vi "Dashboard Main.vi"() -> ()   [LabVIEW 2014]
uses:
  <vilib>/event_ctls.llb/eventvkey.ctl
  <vilib>/Rock Robotics/WPI/Dashboard/WPI_DashboardLogging Global.vi
  <vilib>/Utility/config.llb/Write Key (String).vi
  <vilib>/Utility/config.llb/Write Key (I32).vi
  <vilib>/Utility/file.llb/Write To Spreadsheet File (DBL).vi
  <vilib>/Utility/config.llb/NI_LVConfig.lvlib
panel:
  out "Camera Image 2":T1(plugin-control)
  in  "TCP":refnum<k5>
  in  "Vision":u16(ring) items=["Camera Off", "USB Camera SW", "USB Camera HW", "IP Camera"]
  out "Image Message":string="Timeout in Camera Communications"
  in  "Dashboard Tab":T2(tab)
  in  "DUD CAM":T3={"Frame Rate"=30, "Compression"=30, "Size"=1} {"Frame Rate" scale=1.0..30.0; "Size" items=["640x480", "320x240", "160x120"]}
  out "MotorChart R":cluster{"Numeric":dbl, "Numeric":dbl}(graph)
  out "MotorChart L":T4(graph)
  out "MotorSliders R":cluster{"MotorSlide1":dbl, "MotorSlide2":dbl} {"MotorSlide2" scale=-1.0..1.0 scale format="%#_2e"; "MotorSlide1" scale=-1.0..1.0 scale format="%#_2e"}
  out "MotorSliders L":T5 {"MotorSlide4 2" scale=0.0..14.0 scale format="%#_2e"; "MotorSlide2" scale=-1.0..1.0 scale format="%#_2e"; "MotorSlide1" scale=-1.0..1.0 scale format="%#_2e"}
  out "Gyro":dbl(knob) scale=0.0..360.0
  out "JS1 Z":dbl(slide) scale=-1.0..1.0 scale format="%#_2e"
  out "JS1 Graph":cluster{"X":dbl, "Y":dbl}[](graph)
  out "JS1 Buttons":T6
  out "JS2 Z":dbl(slide) scale=-1.0..1.0 scale format="%#_2e"
  out "JS2 Graph":cluster{"X":dbl, "Y":dbl}[](graph)
  out "JS2 Buttons":T6
  out "Mode":T7(ring)=enum."Auto Disabled"
  in  "DB Camera Config":bool
  in  "Big Cam":T3={"Frame Rate"=30, "Compression"=30, "Size"=1} {"Frame Rate" scale=1.0..30.0; "Size" items=["640x480", "320x240", "160x120"]}
  in  "Small Cam":T3={"Frame Rate"=30, "Compression"=30, "Size"=1} {"Frame Rate" scale=1.0..30.0; "Size" items=["640x480", "320x240", "160x120"]}
  in  "CamPow":bool
  in  "Toggle View":bool
  in  "Rec Mode":enum32{"Stop", "Record", "Playback"}(radio)
  out "Mbps 2":bool
  out "Mbps":dbl format="%#.1g"
  out "fps":dbl format="%#.1g"
  out "Mbps 4":bool
  out "Mbps 3":dbl format="%#.1g"
  out "fps 2":dbl format="%#.1g"
  out "Camera Addr":string
  in  "DB/String 9":string
  in  "DB/String 8":string
  in  "DB/String 7":string
  in  "DB/String 6":string
  in  "DB/String 5":string
  in  "DB/String 4":string
  in  "DB/String 3":string
  in  "DB/String 2":string
  in  "DB/String 1":string
  in  "DB/String 0":string
  in  "DB/Slider 0":dbl(slide) scale=0.0..5.0
  in  "DB/Slider 1":dbl(slide) scale=0.0..5.0
  in  "DB/Slider 2":dbl(slide) scale=0.0..5.0
  in  "DB/Slider 3":dbl(slide) scale=0.0..5.0
  out "DB/LED 3":bool
  out "DB/LED 2":bool
  out "DB/LED 1":bool
  out "DB/LED 0":bool
  in  "DB/Button 3":bool
  in  "DB/Button 2":bool
  in  "DB/Button 1":bool
  in  "DB/Button 0":bool caption="New Name"
  in  "Elevator Go":bool
  in  "Elevator Height":sgl(slide) step=1 scale=0.0..5.0 scale format="%#1.1g"
  in  "Sub Tote":bool
  in  "Add Tote":bool
  out "Tote Count":dbl
  in  "Manual Control":bool
  in  "Winch Cim 2":dbl(slide) scale=-1.0..1.0
  in  "Winch Cim 1":dbl(slide) scale=-1.0..1.0
  in  "Ejector Motor":dbl(slide) scale=-1.0..1.0
  in  "End Effector Motor 1":dbl(slide) scale=-1.0..1.0
  in  "End Effector Motor 2":dbl(slide) scale=-1.0..1.0
  in  "Left Drive Motor":dbl(slide) scale=-1.0..1.0
  in  "Right Drive Motor":dbl(slide) scale=-1.0..1.0
  in  "Test Slider":dbl(slide) scale=0.0..100.0 scale format="%#_3g"
  in  "On/Off":bool caption="Solenoid"
  in  "Test Name":u16(ring) items=["Select the test to run...", "Example Test", "-------------------------------", "List of tests is built in robot code.", "Replace with your own automated tests."]
  in  "Test Tree":string(tree)
  in  "Motor":cluster{"Value":dbl, "Enable":bool} {"Value" scale=-1.0..1.0 scale format="%#_3g"}
  out "Progress":T8 {"Test Progress" scale=0.0..100.0}
  in  "Rev/Fwd":cluster{"Forward":bool, "Reverse":bool}
  in  "Test Ring":u16(ring) items=["Monochrome", "Color"]
  in  "Listbox":i32(listbox)
  out "Tree":string(tree)
  in  "Save To":path
  in  "Export To File":bool
  out "Camera Image":T1(plugin-control)
  out "Boolean":bool
  # "Left"
  # "Front"
  # "Right"
  # "Battery"
  # "Big Cam"
  # "Small Cam"
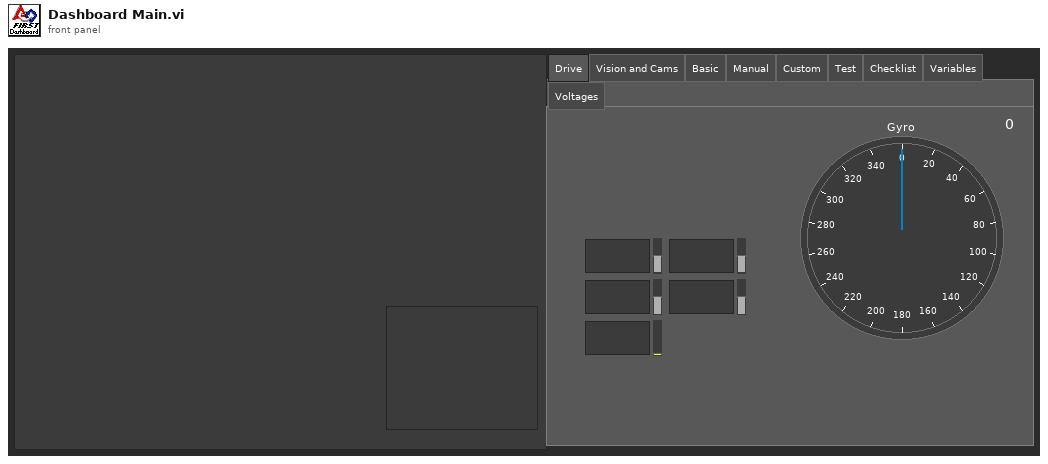
[diagram p1: front panel]
types:
  T1 = typedef "IMAQ Image.ctl" = refnum<image>
  T2 = enum32{"Drive", "Vision and Cams", "Basic", "Manual", "Custom", "Test", "Checklist", "Variables", "Voltages"}
  T3 = cluster{"Frame Rate":i32, "Compression":i32, "Size":u16}
  T4 = cluster{"Numeric":dbl, "Numeric":dbl, "Battery V":dbl}
  T5 = cluster{"MotorSlide1":dbl, "MotorSlide2":dbl, "MotorSlide4 2":dbl}
  T6 = cluster{bool, bool, bool, bool, bool, bool, bool, bool, bool, bool, bool, bool}
  T7 = enum8{"Tele-Op Disabled", "Tele-Op Enabled", "Auto Disabled", "Auto Enabled", "Test Disabled", "Test Enabled", "Disconnected", "No Code", "E-Stop"}
  T8 = cluster{"Test Progress":u8, "Test Progress Text":string}
  T9 = typedef "Image Type" = u32
  T10 = enum32{"Drive", "Basic", "Custom", "Test", "Checklist", "Variables"}
  T11 = cluster{"Camera Image":refnum<vi>, "Dashboard Tab":refnum<vi>, "Boolean":refnum<vi>, "Vision":refnum<vi>, "Rec Mode":refnum<vi>, "Test Slider":refnum<vi>, "On/Off ":refnum<vi>, "Test Ring":refnum<vi>, "Rev/Fwd":refnum<vi>, "Test Name":refnum<vi>, "Motor":refnum<vi>, "Progress":refnum<vi>, "CheckList":refnum<vi>, "Tree":refnum<vi>, "Test Tree":refnum<vi>}
  T12 = cluster{"Error Strings":string, "Disable Counts":cluster{u16, u16}, "Rail Faults":cluster{u16, u16, u16}, "Robot IP":string, "DB Mode":u8, "Event Info":cluster{"Name":string, "Type":u8, "Number":u16, "Replay":u8}, "Camera Addr":string}
  T13 = cluster{"Storage":cluster{"Disk Free":u64, "RAM Block":u32, "RAM free":u32}, "CPU Utilization":cluster{"CPU % ISR":sgl, "CPU % Time Crit":sgl, "CPU % Timed Str":sgl, "CPU % High":sgl, "CPU % Above":sgl, "CPU % Normal":sgl, "CPU % Low":sgl}, "CAN":cluster{"% Bus Utilization":sgl, "Bus Off Cnt":u32, "TX_FIFO Full Cnt":u32, "Receive Error Cnt":u8, "Transmit Error Cnt":u8}, "HID":cluster{"HID Outputs":u32, "Rumble Low":u16, "Rumble High":u16}[]}
  T14 = cluster{"Status bits":cluster{"Test Mode":bool, "Autonomous":bool, "Enabled":bool, "Code Start":bool, "Brownout":bool, "Reserved 2":bool, "Reserved 3":bool, "E-Stop":bool}, "Code Trace":cluster{"Disabled":bool, "TeleOp":bool, "Auto":bool, "Test":bool}, "Controller Type":enum16{"unknown", "cRIO", "roboRio"}, "Code?":enum16{"unknown", "noCode", "code"}, "Battery V":dbl}
  T15 = cluster{"Control Bits":cluster{"TestMode":bool, "Autonomous":bool, "Enabled":bool, "FMS Present":bool, bool, bool, bool, "E-Stop":bool}, "Team Station ":u8, "Countdown":sgl, "Joystick Values":cluster{"Axes":dbl[], "Buttons":bool[], "POVs":i16[]}[]}
  T16 = cluster{"Axes":dbl[], "Buttons":bool[], "POVs":i16[]}[]
  T17 = cluster{"Axes":dbl[], "Buttons":bool[], "POVs":i16[]}
  T18 = cluster{"Buttons[0]":bool, "Buttons[1]":bool, "Buttons[2]":bool, "Buttons[3]":bool, "Buttons[4]":bool, "Buttons[5]":bool, "Buttons[6]":bool, "Buttons[7]":bool, "Buttons[8]":bool, "Buttons[9]":bool, "Buttons[10]":bool, "Buttons[11]":bool}
  T19 = typedef "NI_LVConfig.lvlib/Config Data RefNum.ctl" = refnum<k1>
  T20 = cluster{"Operation":enum16{"Update", "Clear"}, "Color Box":u32}[]
  T21 = typedef "eventvkey.ctl" = enum16{"ASCII", "Enter", "Return", "Shift", "Ctrl", "Alt", "Cmd", "Opt", "Caps", "NumLock", "Clear", "Break", "Up", "Down", "Left", "Right", "Insert", "Delete", "Home", "End", "PageUp", "PageDown", "Escape", "Help", "Pause", "ScrollLock", "F1", "F2", "F3", "F4", "F5", "F6", "F7", "F8", "F9", "F10", "F11", "F12", "F13", "F14", "F15", "F16", "F17", "F18", "F19", "F20", "F21", "F22", "F23", "F24", "Play", "VolumeUp", "VolumeDown", "Mute", "Two Byte Char"}
  T22 = cluster{"Image Size":bool, "Image Type":bool, "Pixel Value":bool, "ROI Information":bool, "Zoom Factor":bool}
  T23 = enum8{"Enabled", "Disabled", "Disabled and Grayed Out"}
  T24 = cluster{"Operation":enum16{"Update", "Clear"}, "Color Box":u32}
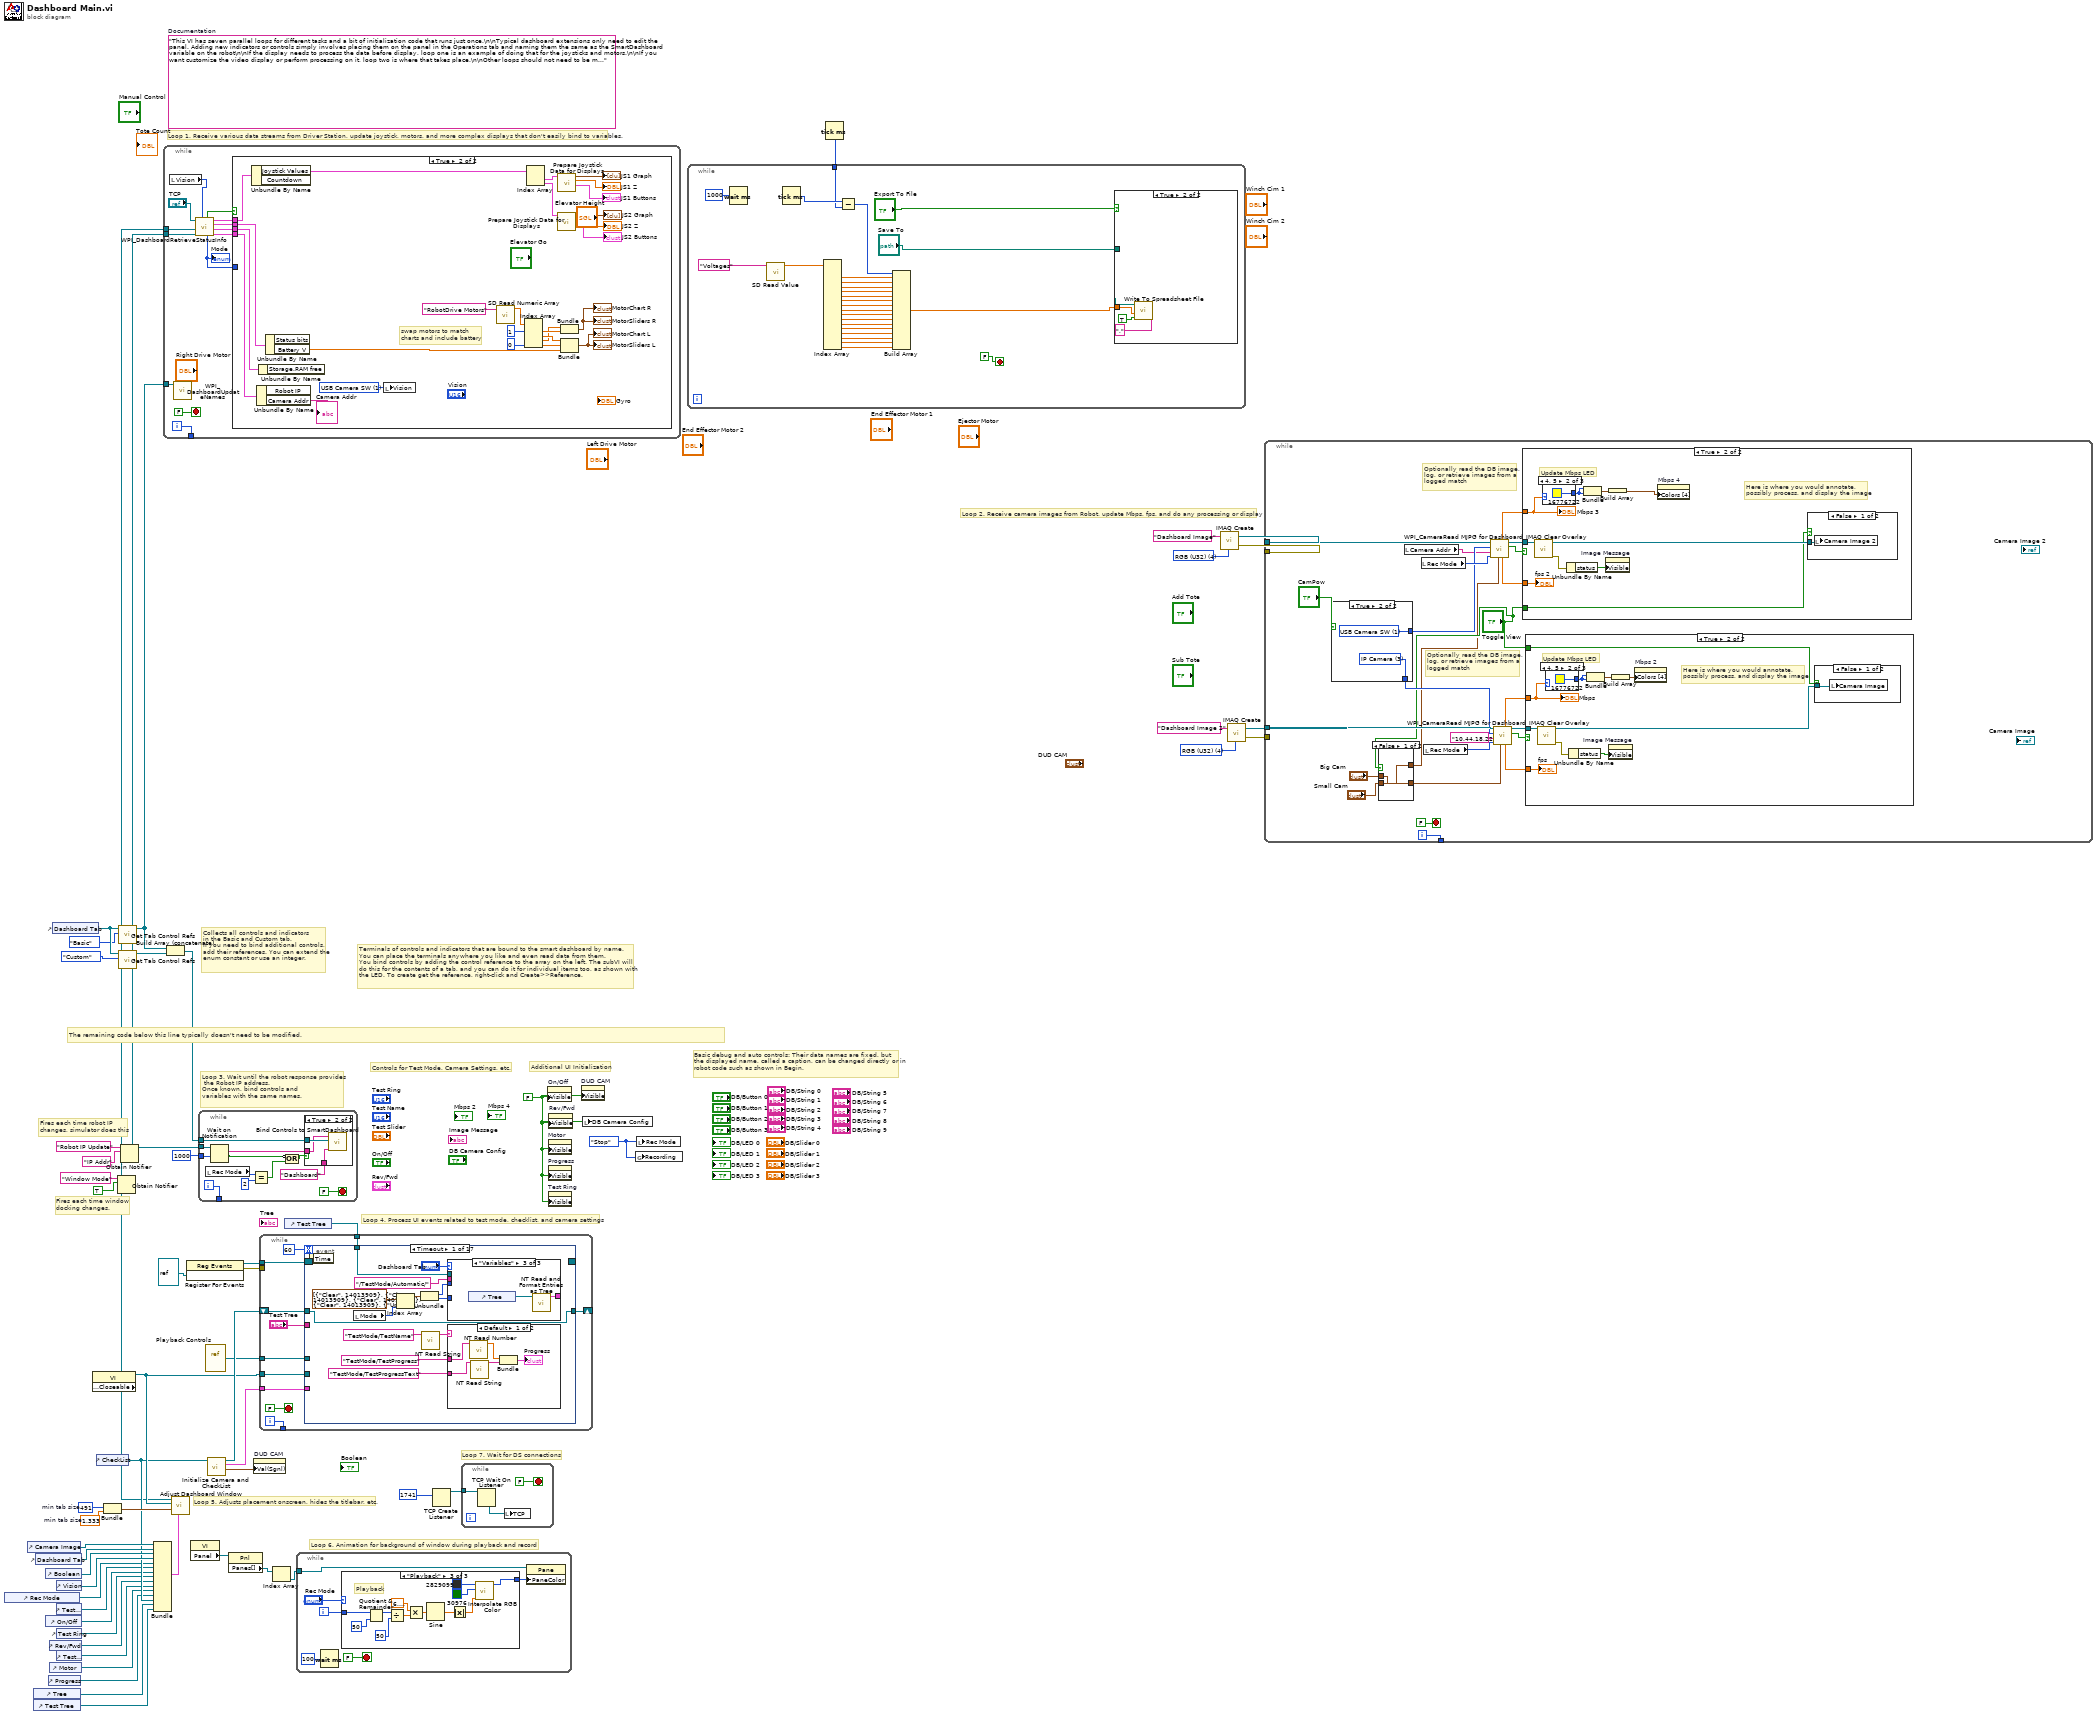
[diagram p0: block diagram]
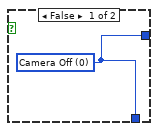
[diagram p3: hidden frame]
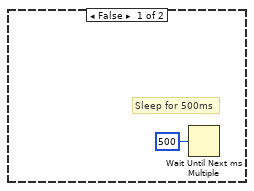
[diagram p4: hidden frame]
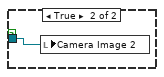
[diagram p5: hidden frame]
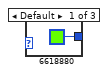
[diagram p6: hidden frame]
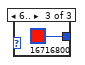
[diagram p7: hidden frame]
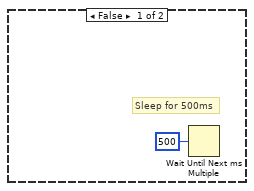
[diagram p8: hidden frame]
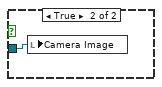
[diagram p9: hidden frame]
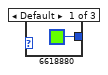
[diagram p10: hidden frame]
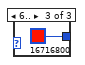
[diagram p11: hidden frame]
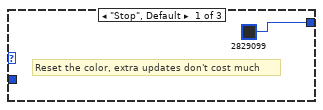
[diagram p14: hidden frame]
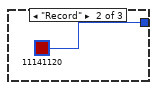
[diagram p15: hidden frame]
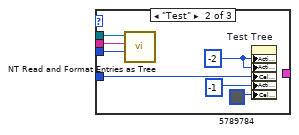
[diagram p18: hidden frame]
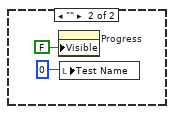
[diagram p19: hidden frame]
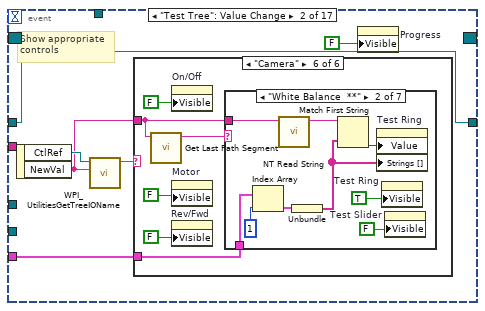
[diagram p20: hidden frame]
diagram:
  w7 = T9 4 items=["Grayscale (U8)", "Grayscale (I16)", "Grayscale (SGL)", "Complex (CSG)", "RGB (U32)", "HSL (U32)", "RGB (U64)"] ("Image Type")
  w32 = 491  # min tab size
  w31 = 1.333  # min tab size
  w3 = enum32{"Stop", "Record", "Playback"}."Stop" ("Rec Mode")
  w14 = FALSE ("Visible")
  (unwired) "This VI has seven parallel loops for different tasks and a bit of initialization code that runs just once.\n\nTypical dashboard extensions only need to edit the panel. Adding new indicators or controls simply involves placing them on the panel in the Operations tab and naming them the same as the SmartDashboard variable on the robot\n\nIf the display needs to process the data before display, loop one is an example of doing that for the joysticks and motors.\n\nIf you want customize the video display or perform processing on it, loop two is where that takes place.\n\nOther loops should not need to be modified. They are pretty standard, and document the task they perform."  # Documentation
  w57 = T9 4 items=["Grayscale (U8)", "Grayscale (I16)", "Grayscale (SGL)", "Complex (CSG)", "RGB (U32)", "HSL (U32)", "RGB (U64)"] ("Image Type")
  # "Loop 7. Wait for DS connections"
  # "Basic debug and auto controls: Their data names are fixed, but\nthe displayed name, called a caption, can be changed directly or in\nrobot code such as shown in Begin."
  # "Controls for Test Mode, Camera Settings, etc."
  # "Additional UI Initialization"
  # "Loop 6. Animation for background of window during playback and record"
  # "Fires each time robot IP\nchanges, simulator does this"
  # "Fires each time window\ndocking changes."
  # "Collects all controls and indicators\nin the Basic and Custom tab.\nIf you need to bind additional controls,\nadd their references. You can extend the\nenum constant or use an integer."
  # "The remaining code below this line typically doesn't need to be modified."
  # "Loop 4. Process UI events related to test mode, checklist, and camera settings"
  # "Terminals of controls and indicators that are bound to the smart dashboard by name.\nYou can place the terminals anywhere you like and even read data from them.\nYou bind controls by adding the control reference to the array on the left. The subVI will\ndo this for the contents of a tab, and you can do it for individual items too, as shown with\nthe LED. To create get the reference, right-click and Create>>Reference."
  # "Loop 3. Wait until the robot response provides\n the Robot IP address.\nOnce known, bind controls and\nvariables with the same names."
  # "Loop 5. Adjusts placement onscreen, hides the titlebar, etc."
  # "Loop 1. Receive various data streams from Driver Station, update joystick, motors, and more complex displays that don't easily bind to variables."
  # "Loop 2. Receive camera images from Robot, update Mbps, fps, and do any processing or display"
  n1 = control-ref of="Rec Mode"() -> (w20:refnum<vi>)
  n2 = control-ref of="Camera Image"() -> (w35:refnum<vi>)
  n3 = control-ref of="Tree"() -> (w24:refnum<vi>)
  n4 = control-ref of="Test Tree"() -> (w23:refnum<vi>)
  n5 = control-ref of="Dashboard Tab"() -> (w34:refnum<vi>)
  n6 = control-ref of="Boolean"() -> (w29:refnum<vi>)
  n7 = control-ref of="On/Off"() -> (w18:refnum<vi>)
  n8 = control-ref of="Progress"() -> (w15:refnum<vi>)
  n9 = control-ref of="Rev/Fwd"() -> (w16:refnum<vi>)
  n10 = control-ref of="Motor"() -> (w21:refnum<vi>)
  n11 = control-ref of="Dashboard Tab"() -> (w38:refnum<vi>)
  n12 = control-ref of="Test Slider"() -> (w19:refnum<vi>)
  n13 = control-ref of="Vision"() -> (w33:refnum<vi>)
  n14 = control-ref of="Test Ring"() -> (w17:refnum<vi>)
  n15 = control-ref of="Test Name"() -> (w22:refnum<vi>)
  n16 = property class="VI" props=["Front Panel.Closeable"]() -> (reference out=w39:refnum<vi>)  [unwired: 2 in, 2 out]
  n17 = control-ref of="CheckList"() -> (w25:refnum<vi>)
  n18 = Bundle("min tab size"=w32, "min tab size"=w31) -> (w30:cluster{"min tab size":i32, "min tab size":dbl})  [unwired: 1 in]
  n19 = Obtain Notifier(name (unnamed)="Window Mode", notification data type=TRUE) -> (notifier out=w11:refnum<notifier>)  [unwired: 2 in, 2 out]
  n20 = call <vilib>:"Get Tab Control Refs.vi"("Page Index"=T10."Basic" ("Dashboard Tab"), "TabControl in"=w38) -> ("ControlsOnPage"=w12:refnum<vi>[])  [unwired: 9 in]
  n21 = call <vilib>:"Get Tab Control Refs.vi"("Page Index"=T10."Custom" ("Dashboard Tab"), "TabControl in"=w38) -> ("ControlsOnPage"=w37:refnum<vi>[])  [unwired: 9 in]
  n22 = Obtain Notifier(name (unnamed)="Robot IP Update", notification data type="IP Addr" ("name (unnamed)")) -> (notifier out=w13:refnum<notifier>)  [unwired: 2 in, 2 out]
  n23 = Bundle("Camera Image"=w35, "Dashboard Tab"=w34, "Boolean"=w29, "Vision"=w33, "Rec Mode"=w20, "Test Slider"=w19, "On/Off"=w18, "Test Ring"=w17, "Rev/Fwd"=w16, "Test Name"=w22, "Motor"=w21, "Progress"=w15, "CheckList"=w25, "Tree"=w24, "Test Tree"=w23) -> (w26:T11)  [unwired: 1 in]
  n24 = while {
    tunnel: [w69] -> _
    tunnel: w13 -> [w63]
    tunnel: w12 -> [w62]
    tunnel: w11 -> [w58]
    i -> [w69]
    stop <- FALSE stop-if-true
    n25 = local read "Vision"() -> (w60:u16)
    n26 = call <vilib>:"WPI_DashboardUpdateNames.vi"("Controls on Tab"=w62) -> ()  [unwired: 11 in]
    n27 = call <vilib>:"WPI_DashboardRetrieveStatusInfo.vi"("Vision"=w60, "Binding Refnum"=w63, "Window Mode Notifier"=w58, "TCP Cnx"="TCP") -> ("Power and Errors"=w64:T12, "Robot Metrics"=w67:T13, "Status Info"=w68:T14, "Control Info"=w65:T15, "Robot Mode"=w61:T7, "Process?"=w66:bool)  [unwired: 2 in]
    "Mode" <- w61
    n28 = case shown="True" w66 {
      tunnel: w68 -> [_ w96]
      tunnel: w67 -> [_ w95]
      tunnel: w65 -> [_ w94]
      tunnel: w64 -> [_ w93]
      tunnel: w61 -> [_ _]
      frame False {
      }
      frame True {
        w72 = u16 1 items=["Camera Off", "USB Camera SW", "USB Camera HW", "IP Camera"] ("Vision")
        # "swap motors to match\ncharts and include battery"
        n29 = Unbundle By Name(w94) -> ("Joystick Values"=w81:T16)  [unwired: 1 out]
        n30 = Unbundle By Name(w93) -> ("Camera Addr"=→"Camera Addr":string)  [unwired: 1 out]
        n31 = Unbundle By Name(w95) -> ()  [unwired: 1 out]
        n32 = Unbundle By Name(w96) -> ("Battery V"=w82:dbl)  [unwired: 1 out]
        n33 = local write "Vision"(w72) -> ()
        n34 = call <vilib>:"SD Read Numeric Array.vi"("Name"="RobotDrive Motors") -> ("Numeric Array"=w84:dbl[])  [unwired: 8 in, 2 out]
        n35 = Index Array(array=w84, index #1=1, index #4=0) -> (element #1=w88:dbl, element #2=w89:dbl, element #3=w87:dbl, element #4=w92:dbl)  [unwired: 2 in]
        n36 = Index Array(array=w81) -> (element #1=w80:T17, element #2=w76:T17)  [unwired: 2 in]
        n37 = call "Prepare Joystick Data for Displays.vi"("Joystick Values"=w76) -> ("Buttons"=→"JS2 Buttons":T18, "Z Axis"=→"JS2 Z":dbl, "Cartesian Data"=→"JS2 Graph":cluster{"X axis":dbl, "X axis":dbl}[])  [unwired: 8 in]
        n38 = call "Prepare Joystick Data for Displays.vi"("Joystick Values"=w80) -> ("Buttons"=→"JS1 Buttons":T18, "Z Axis"=→"JS1 Z":dbl, "Cartesian Data"=→"JS1 Graph":cluster{"X axis":dbl, "X axis":dbl}[])  [unwired: 8 in]
        n39 = Bundle("Numeric"=w87, "Numeric"=w88) -> (→"MotorChart R" →"MotorSliders R":cluster{"Numeric":dbl, "Numeric":dbl})  [unwired: 1 in]
        n40 = Bundle("Numeric"=w89, "Numeric"=w92, "Battery V"=w82) -> (→"MotorChart L" →"MotorSliders L":T4)  [unwired: 1 in]
      }
    }
  }
  n41 = Build Array (concatenate)(w12, w37) -> (w36:refnum<vi>[])
  n42 = call "Adjust Dashboard Window.vi"("Sizing Refnums"=w26, "Size Constraints"=w30, "VI"=w39, "Notifier in"=w11) -> ()  [unwired: 8 in]
  n43 = register-events(refnum<vi> refnum) -> (reference out=w43:refnum<event-registration>, error out=w42:errorcluster)  [unwired: 2 in]
  n44 = property class="VI"() -> ("Panel"=w46:refnum<vi>)  [unwired: 2 in, 2 out]
  n45 = while {
    tunnel: w36 -> [w108]
    tunnel: w13 -> [w106]
    tunnel: [w104] -> _
    tunnel: u32 1000 ("milliseconds to wait") -> [w103]
    i -> [w104]
    stop <- FALSE stop-if-true
    n46 = local read "Rec Mode"() -> (w99:enum32{"Stop", "Record", "Playback"})
    n47 = Wait on Notification(notifier=w106, timeout in ms (-1)=w103) -> (notification=w105:string, timed out?=w101:bool)  [unwired: 2 in, 2 out]
    n48 = Equal?(x=w99, y=u16 2 ("Rec Mode")) -> (x = y?=w100:bool)
    n49 = Compound Arithmetic op=OR(invert w101, w100) -> (w102:bool)
    n50 = case shown="True" w102 {
      tunnel: w108 -> [_ w111]
      tunnel: w105 -> [_ w110]
      tunnel: "Dashboard" -> [_ w109]
      frame False {
      }
      frame True {
        n51 = call <vilib>:"Bind Controls to SmartDashboard.vi"("Client Name"=w109, "Bound Control Refs"=w111, "Server IP Address"=w110) -> ()  [unwired: 9 in]
      }
    }
  }
  n52 = vi-ref "Playback Controls.vi"() -> (w44:refnum<vi>)
  n53 = call "Initialize Camera and CheckList.vi"("ListBox in"=w25) -> ("Cluster"=w50:cluster{"value":i32, "value":i32, "index":i32}, "Array"=w51:cluster{string[]}[], "File Refnum"=w49:T19)  [unwired: 8 in]
  n54 = property class="Pnl"(reference=w46) -> ("Panes[]"=w47:refnum<vi>[])  [unwired: 1 in, 2 out]
  n55 = property on="DUD CAM" class="Clust (strict)"("Val(Sgnl)"=w50) -> ()  [unwired: 2 in, 2 out]
  n56 = Index Array(array=w47) -> (element=w45:refnum<vi>)  [unwired: 1 in]
  n57 = control-ref of="Test Tree"() -> (w48:refnum<vi>)
  n58 = while {
    tunnel: w51 -> [w119]
    shift-right: [w118] -> _
    shift-left: w49 -> [w117]
    tunnel: [w116] -> _
    tunnel: w48 -> [w115]
    tunnel: w44 -> [w114]
    tunnel: w43 -> [w113]
    tunnel: w42 -> [_]
    tunnel: w39 -> [w112]
    i -> [w116]
    stop <- FALSE stop-if-true
    n59 = event shown="[0] Timeout" {
      selector: w113 -> [_ _ _ _ _ _ _ _ _ _ _ _ _ _ _ _ _]
      dyn-events: [_ _ _ _ _ _ _ _ _ _ _ _ _ w357 _ _ _] -> _
      timeout: u32 60 ("milliseconds to wait") -> [_ _ _ _ _ _ _ _ _ _ _ _ _ _ _ _ _]
      tunnel: w115 -> [w131 _ _ _ _ _ _ _ _ _ _ _ _ _ _ _ _]
      tunnel: "Test Tree" -> [_ _ _ _ _ _ _ _ w326 w334 w336 w340 w348 _ _ _ _]
      tunnel: w119 -> [_ w153 _ _ _ _ w290 w320 _ _ _ _ _ _ _ _ _]
      tunnel: [w127 w152 w251 w256 w264 w276 w289 w313 w325 w332 w335 w339 w347 w359 w373 w374 w384] -> w118
      tunnel: w117 -> [w127 w152 w251 w256 w264 w276 w288 w313 w325 w332 w335 w339 w347 w359 w373 w374 w384]
      tunnel: w114 -> [_ _ _ _ _ _ _ _ _ _ _ _ _ w360 _ w377 _]
      tunnel: w112 -> [_ _ _ _ _ _ _ _ _ _ _ _ _ w355 _ _ _]
      event Timeout {
        n60 = event-data() -> ()  [unwired: 1 in, 1 out]
        n61 = local read "Mode"() -> (w130:T7)
        n62 = Index Array(array=T20 [{"Operation"=enum."Clear", "Color Box"=14013909}, {"Operation"=enum."Clear", "Color Box"=14013909}, {"Operation"=enum."Clear", "Color Box"=14013909}, {"Operation"=enum."Clear", "Color Box"=14013909}, {"Operation"=enum."Update", "Color Box"=14013909}, {"Operation"=enum."Update", "Color Box"=16777215}, {"Operation"=enum."Clear", "Color Box"=14013909}, {"Operation"=enum."Clear", "Color Box"=14013909}, {"Operation"=enum."Clear", "Color Box"=14013909}], index=w130) -> (element=w125:T24)
        n63 = Unbundle(w125) -> ("Operation"=w124:enum16{"Update", "Clear"}, "Color Box"=w123:u32)
        n64 = call <vilib>:"NT Read String.vi"("Name"="TestMode/TestName") -> ("String"=w134:string)  [unwired: 9 in, 1 out]
        n65 = case shown="\"Variables\"" "Dashboard Tab" {
          tunnel: w131 -> [_ w142 _]
          tunnel: "/TestMode/Automatic/" ("Name Pattern") -> [_ w141 _]
          tunnel: w124 -> [_ w140 _]
          tunnel: [_ _ w144] -> _
          tunnel: w123 -> [_ w136 _]
          frame "Custom", Default {
          }
          frame "Test" {
            w139 = -2 ("Active Item:Row Number")
            n66 = call <vilib>:"NT Read and Format Entries as Tree.vi"("Operation"=w140, "Name Pattern"=w141, "Tree Refnum"=w142) -> ()  [unwired: 7 in, 2 out]
            n67 = property on="Test Tree" class="Tree (strict)"("Active Item Row Number"=w139, "ActiveColNum"=w139, "CellBG"=w136, "Active Item Row Number"=-1 ("Active Item:Row Number"), "CellBG"=u32 5789784 ("Color Box")) -> ()  [unwired: 2 in, 2 out]
          }
          frame "Variables" {
            n68 = control-ref of="Tree"() -> (w143:refnum<vi>)
            n69 = call <vilib>:"NT Read and Format Entries as Tree.vi"("Tree Refnum"=w143) -> ("Formatted Strings"=w144:cluster{"Name":string, "Value":string}[])  [unwired: 9 in, 1 out]
          }
        }
        n70 = case shown="Default" w134 {
          tunnel: "TestMode/TestProgress" ("Name") -> [w146 _]
          tunnel: "TestMode/TestProgressText" ("Name") -> [w145 _]
          frame Default {
            n71 = call <vilib>:"NT Read Number.vi"("Name"=w146) -> ("Numeric"=w147:dbl)  [unwired: 9 in, 1 out]
            n72 = call <vilib>:"NT Read String.vi"("Name"=w145) -> ("String"=w148:string)  [unwired: 9 in, 1 out]
            n73 = Bundle("Numeric"=w147, "String"=w148) -> (→"Progress":cluster{"Numeric":dbl, "String":string})  [unwired: 1 in]
          }
          frame "" {
            n74 = property on="Progress" class="Clust (strict)"("Visible"=FALSE) -> ()  [unwired: 2 in, 2 out]
            n75 = local write "Test Name"(u16 0) -> ()
          }
        }
      }
      event "Test Tree": Value Change {
        # "Show appropriate\ncontrols"
        n76 = event-data() -> ("CtlRef"=w156:refnum<vi>, "NewVal"=w154:string)  [unwired: 1 in]
        n77 = call <vilib>:"WPI_UtilitiesGetTreeIOName.vi"("NewVal"=w154, "TreeControl in"=w156) -> ("I/O Name"=w157:string)  [unwired: 9 in]
        n78 = case shown="\"Camera\"" w157 {
          selector: w157 -> [_ w164 _ w182 w191 _]
          tunnel: w154 -> [_ _ w179 w181 _ w198]
          tunnel: w153 -> [_ _ _ _ _ w197]
          frame Default {
            w159 = FALSE ("Visible")
            w158 = FALSE ("Visible")
            n79 = property on="Motor" class="Clust (strict)"("Visible"=w158) -> ()  [unwired: 2 in, 2 out]
            n80 = property on="Test Ring" class="Ring (strict)"("Visible"=w158) -> ()  [unwired: 2 in, 2 out]
            n81 = property on="Rev/Fwd" class="Clust (strict)"("Visible"=w159) -> ()  [unwired: 2 in, 2 out]
            n82 = property on="On/Off" class="Bool (strict)"("Visible"=w159) -> ()  [unwired: 2 in, 2 out]
            n83 = property on="Test Slider" class="Slide (strict)"("Visible"=w159) -> ()  [unwired: 2 in, 2 out]
          }
          frame "Motor", "PWM" {
            w165 = FALSE ("Visible")
            n84 = case shown="\"Motor\", Default" w164 {
              tunnel: [1.0 ("Value") -1.0 ("Value")] -> w163
              tunnel: [255.0 ("Value") 1.0 ("Value")] -> w162
              tunnel: [128.0 ("Value") 0.0 ("Value")] -> w161
              tunnel: [64.0 ("Value") 0.5 ("Value")] -> w160
              frame "PWM" {
              }
              frame "Motor", Default {
              }
            }
            n85 = property on="Motor" class="Clust (strict)"("Visible"=TRUE) -> ()  [unwired: 2 in, 2 out]
            n86 = property on="Value" class="Slide (strict)"("Value"=w161, "Scale.Minimum"=w163, "Scale.Maximum"=w162, "Scale.Increment"=w160) -> ()  [unwired: 2 in, 2 out]
            n87 = property on="On/Off" class="Bool (strict)"("Visible"=w165) -> ()  [unwired: 2 in, 2 out]
            n88 = property on="Test Slider" class="Slide (strict)"("Visible"=w165) -> ()  [unwired: 2 in, 2 out]
            n89 = property on="Test Ring" class="Ring (strict)"("Visible"=w165) -> ()  [unwired: 2 in, 2 out]
            n90 = property on="Rev/Fwd" class="Clust (strict)"("Visible"=w165) -> ()  [unwired: 2 in, 2 out]
          }
          frame "Servo" {
            w177 = FALSE ("Visible")
            n91 = call <vilib>:"NT Read Number.vi"("Name"=w179) -> ("Numeric"=w178:dbl)  [unwired: 9 in, 1 out]
            n92 = property on="Test Slider" class="Slide (strict)"("Visible"=TRUE, "Scale.Maximum"=170.0 ("Scale.Range:Maximum")) -> ()  [unwired: 2 in, 2 out]
            n93 = local write "Test Slider"(w178) -> ()
            n94 = property on="Motor" class="Clust (strict)"("Visible"=w177) -> ()  [unwired: 2 in, 2 out]
            n95 = property on="Rev/Fwd" class="Clust (strict)"("Visible"=w177) -> ()  [unwired: 2 in, 2 out]
            n96 = property on="On/Off" class="Bool (strict)"("Visible"=w177) -> ()  [unwired: 2 in, 2 out]
            n97 = property on="Test Ring" class="Ring (strict)"("Visible"=w177) -> ()  [unwired: 2 in, 2 out]
          }
          frame "Relay", "Solenoid" {
            w180 = FALSE ("Visible")
            n98 = property on="Motor" class="Clust (strict)"("Visible"=w180) -> ()  [unwired: 2 in, 2 out]
            n99 = property on="Test Slider" class="Slide (strict)"("Visible"=w180) -> ()  [unwired: 2 in, 2 out]
            n100 = Search and Replace String(input string=w181, search string="/Value  **", replace string="/Direction") -> (result string=w187:string)  [unwired: 5 in, 3 out]
            n101 = property on="Test Ring" class="Ring (strict)"("Visible"=w180) -> ()  [unwired: 2 in, 2 out]
            n102 = call <vilib>:"NT Read String.vi"("Name"=w187) -> ("String"=w185:string)  [unwired: 9 in, 1 out]
            n103 = Equal?(x="Both directions", y=w185) -> (x = y?=w183:bool)
            n104 = Not(x=w183) -> (.not. x?=w184:bool)
            n105 = property on="Rev/Fwd" class="Clust (strict)"("Visible"=w183) -> ()  [unwired: 2 in, 2 out]
            n106 = property on="On/Off" class="Bool (strict)"("Visible"=w184, "Caption.Text"=w182) -> ()  [unwired: 2 in, 2 out]
          }
          frame "Compressor", "Digital Out" {
            w190 = FALSE ("Visible")
            # "Get direction and finish"
            n107 = property on="Motor" class="Clust (strict)"("Visible"=w190) -> ()  [unwired: 2 in, 2 out]
            n108 = property on="Test Slider" class="Slide (strict)"("Visible"=w190) -> ()  [unwired: 2 in, 2 out]
            n109 = property on="Test Ring" class="Ring (strict)"("Visible"=w190) -> ()  [unwired: 2 in, 2 out]
            n110 = property on="On/Off" class="Bool (strict)"("Visible"=TRUE, "Caption.Text"=w191) -> ()  [unwired: 2 in, 2 out]
            n111 = property on="Rev/Fwd" class="Clust (strict)"("Visible"=FALSE) -> ()  [unwired: 2 in, 2 out]
          }
          frame "Camera" {
            n112 = call <vilib>:"Get Last Path Segment.vi"("String in"=w198) -> ("String out"=w199:string)  [unwired: 10 in]
            n113 = property on="On/Off" class="Bool (strict)"("Visible"=FALSE) -> ()  [unwired: 2 in, 2 out]
            n114 = property on="Motor" class="Clust (strict)"("Visible"=FALSE) -> ()  [unwired: 2 in, 2 out]
            n115 = property on="Rev/Fwd" class="Clust (strict)"("Visible"=FALSE) -> ()  [unwired: 2 in, 2 out]
            n116 = case shown="\"White Balance  **\"" w199 {
              tunnel: w198 -> [w205 w214 w223 w232 w241 _ w247]
              tunnel: w197 -> [w203 w211 w220 w229 w238 _ _]
              frame "Size  **" {
                n117 = Index Array(array=w203) -> (element=w202:cluster{string[]})  [unwired: 1 in]
                n118 = call <vilib>:"NT Read String.vi"("Name"=w205) -> ("String"=w204:string)  [unwired: 9 in, 1 out]
                n119 = Unbundle(w202) -> (w200:string[])
                n120 = Match First String(2:w200, 3:w204) -> (0:w201:i32)  [unwired: 1 out]
                n121 = property on="Test Ring" class="Ring (strict)"("Value"=w201, "Strings []"=w200) -> ()  [unwired: 2 in, 2 out]
                n122 = property on="Test Ring" class="Ring (strict)"("Visible"=TRUE) -> ()  [unwired: 2 in, 2 out]
                n123 = property on="Test Slider" class="Slide (strict)"("Visible"=FALSE) -> ()  [unwired: 2 in, 2 out]
              }
              frame "White Balance  **" {
                n124 = Index Array(array=w211, index=1) -> (element=w212:cluster{string[]})
                n125 = call <vilib>:"NT Read String.vi"("Name"=w214) -> ("String"=w213:string)  [unwired: 9 in, 1 out]
                n126 = Unbundle(w212) -> (w209:string[])
                n127 = Match First String(2:w209, 3:w213) -> (0:w208:i32)  [unwired: 1 out]
                n128 = property on="Test Ring" class="Ring (strict)"("Value"=w208, "Strings []"=w209) -> ()  [unwired: 2 in, 2 out]
                n129 = property on="Test Ring" class="Ring (strict)"("Visible"=TRUE) -> ()  [unwired: 2 in, 2 out]
                n130 = property on="Test Slider" class="Slide (strict)"("Visible"=FALSE) -> ()  [unwired: 2 in, 2 out]
              }
              frame "Exposure  **" {
                n131 = Index Array(array=w220, index=2) -> (element=w221:cluster{string[]})
                n132 = call <vilib>:"NT Read String.vi"("Name"=w223) -> ("String"=w222:string)  [unwired: 9 in, 1 out]
                n133 = Unbundle(w221) -> (w217:string[])
                n134 = Match First String(2:w217, 3:w222) -> (0:w218:i32)  [unwired: 1 out]
                n135 = property on="Test Ring" class="Ring (strict)"("Value"=w218, "Strings []"=w217) -> ()  [unwired: 2 in, 2 out]
                n136 = property on="Test Ring" class="Ring (strict)"("Visible"=TRUE) -> ()  [unwired: 2 in, 2 out]
                n137 = property on="Test Slider" class="Slide (strict)"("Visible"=FALSE) -> ()  [unwired: 2 in, 2 out]
              }
              frame "Exposure Priority  **" {
                n138 = Index Array(array=w229, index=3) -> (element=w230:cluster{string[]})
                n139 = call <vilib>:"NT Read String.vi"("Name"=w232) -> ("String"=w231:string)  [unwired: 9 in, 1 out]
                n140 = Unbundle(w230) -> (w226:string[])
                n141 = Match First String(2:w226, 3:w231) -> (0:w227:i32)  [unwired: 1 out]
                n142 = property on="Test Ring" class="Ring (strict)"("Value"=w227, "Strings []"=w226) -> ()  [unwired: 2 in, 2 out]
                n143 = property on="Test Ring" class="Ring (strict)"("Visible"=TRUE) -> ()  [unwired: 2 in, 2 out]
                n144 = property on="Test Slider" class="Slide (strict)"("Visible"=FALSE) -> ()  [unwired: 2 in, 2 out]
              }
              frame "Color Enable  **" {
                n145 = Index Array(array=w238, index=4) -> (element=w239:cluster{string[]})
                n146 = call <vilib>:"NT Read String.vi"("Name"=w241) -> ("String"=w240:string)  [unwired: 9 in, 1 out]
                n147 = Unbundle(w239) -> (w235:string[])
                n148 = Match First String(2:w235, 3:w240) -> (0:w236:i32)  [unwired: 1 out]
                n149 = property on="Test Ring" class="Ring (strict)"("Value"=w236, "Strings []"=w235) -> ()  [unwired: 2 in, 2 out]
                n150 = property on="Test Ring" class="Ring (strict)"("Visible"=TRUE) -> ()  [unwired: 2 in, 2 out]
                n151 = property on="Test Slider" class="Slide (strict)"("Visible"=FALSE) -> ()  [unwired: 2 in, 2 out]
              }
              frame Default {
                n152 = property on="Test Ring" class="Ring (strict)"("Visible"=FALSE) -> ()  [unwired: 2 in, 2 out]
                n153 = property on="Test Slider" class="Slide (strict)"("Visible"=FALSE) -> ()  [unwired: 2 in, 2 out]
              }
              frame "Brightness  **", "Color Level  **", "Compression  **", "FPS  **", "Sharpness  **" {
                n154 = call <vilib>:"NT Read Number.vi"("Name"=w247) -> ("Numeric"=w246:dbl)  [unwired: 9 in, 1 out]
                n155 = local write "Test Slider"(w246) -> ()
                n156 = property on="Test Slider" class="Slide (strict)"("Visible"=TRUE, "Scale.Maximum"=100.0 ("Scale.Range:Maximum")) -> ()  [unwired: 2 in, 2 out]
                n157 = property on="Test Ring" class="Ring (strict)"("Visible"=FALSE) -> ()  [unwired: 2 in, 2 out]
              }
            }
          }
        }
        n158 = property on="Progress" class="Clust (strict)"("Visible"=FALSE) -> ()  [unwired: 2 in, 2 out]
      }
      event "Test Name": Mouse Enter {
        # "Populate the ring with the list of tests"
        n159 = event-data() -> ()  [unwired: 1 in, 1 out]
        n160 = call <vilib>:"NT Read String Array.vi"("Name"="TestMode/TestList") -> ("String Array"=w255:string[])  [unwired: 9 in, 1 out]
        n161 = Build Array (concatenate)("Select the test to run...", w255) -> (w254:string[])
        n162 = property on="Test Name" class="Ring (strict)"("Strings []"=w254) -> ()  [unwired: 2 in, 2 out]
      }
      event "Test Name": Value Change {
        w257 = FALSE ("Visible")
        # "Tell the robot the test name to run"
        n163 = event-data() -> ("NewVal"=w261:u16)  [unwired: 1 in]
        n164 = property on="Test Name" class="Ring (strict)"() -> ("Strings []"=w262:string[])  [unwired: 2 in, 2 out]
        n165 = local write "Progress"(T8 {"Test Progress"=0, "Test Progress Text"=""} ("Progress")) -> ()
        n166 = Index Array(array=w262, index=w261) -> (element=w260:string)
        n167 = call <vilib>:"NT Write String.vi"("String"=w260, "Name"="TestMode/TestName") -> ()  [unwired: 9 in, 1 out]
        n168 = property on="Progress" class="Clust (strict)"("Visible"=TRUE) -> ()  [unwired: 2 in, 2 out]
        n169 = property on="Motor" class="Clust (strict)"("Visible"=w257) -> ()  [unwired: 2 in, 2 out]
        n170 = property on="Test Slider" class="Slide (strict)"("Visible"=w257) -> ()  [unwired: 2 in, 2 out]
        n171 = property on="On/Off" class="Bool (strict)"("Visible"=w257) -> ()  [unwired: 2 in, 2 out]
        n172 = property on="Rev/Fwd" class="Clust (strict)"("Visible"=w257) -> ()  [unwired: 2 in, 2 out]
        n173 = property on="Test Ring" class="Ring (strict)"("Visible"=w257) -> ()  [unwired: 2 in, 2 out]
      }
      event "Listbox": Double Click {
        # "Shift clears all"
        # "Update symbols on the listbox"
        n174 = event-data() -> ("PlatMods.Shift"=w265:bool, "Row"=w267:i32)  [unwired: 1 in]
        n175 = case shown="True" w265 {
          tunnel: w267 -> [w271 _]
          tunnel: 1 -> [w270 _]
          frame False {
            n176 = property on="Listbox" class="LstBox (strict)"() -> ("Item Symbols"=w269:i32[])  [unwired: 2 in, 2 out]
            n177 = Replace Array Subset(array=w269, new element=w270, index=w271) -> (w268:i32[])
            n178 = property on="Listbox" class="LstBox (strict)"("Item Symbols"=w268) -> ()  [unwired: 2 in, 2 out]
          }
          frame True {
            w272 = 0 ("Top Row")
            n179 = property on="Listbox" class="LstBox (strict)"() -> ("Number of Rows"=w274:u32)  [unwired: 2 in, 2 out]
            n180 = Initialize Array(0, w274) -> (w273:i32[])
            n181 = property on="Listbox" class="LstBox (strict)"("Top Row"=w272, "Value"=w272, "Item Symbols"=w273) -> ()  [unwired: 2 in, 2 out]
          }
        }
      }
      event "Listbox": Key Down {
        # "Update symbols on the listbox\nLeft and right keys check and uncheck"
        n182 = event-data() -> ("VKey"=w278:T21)  [unwired: 1 in]
        n183 = case shown="\"Left\", \"Right\"" w278 {
          selector: w278 -> [w283 _]
          tunnel: eventvkey."Left" ("VKey") -> [w281 _]
          frame "Left", "Right" {
            n184 = Equal?(x=w281, y=w283) -> (x = y?=w282:bool)
            n185 = Select(t=0, s=w282, f=1) -> (s? t:f=w284:i32)
            n186 = property on="Listbox" class="LstBox (strict)"() -> ("Item Symbols"=w287:i32[])  [unwired: 2 in, 2 out]
            n187 = Replace Array Subset(array=w287, new element=w284, index="Listbox") -> (w286:i32[])
            n188 = property on="Listbox" class="LstBox (strict)"("Item Symbols"=w286) -> ()  [unwired: 2 in, 2 out]
          }
          frame Default {
          }
        }
      }
      event "DB Camera Config": Value Change {
        # "Show or hide the cluster of controls, store in ini file"
        n189 = event-data() -> ("NewVal"=w291:bool)  [unwired: 1 in]
        n190 = case shown="False" w291 {
          tunnel: w290 -> [w300 _]
          tunnel: [w293 w311] -> w289
          tunnel: w288 -> [w292 w311]
          frame False {
            w307 = "Camera"
            w310 = FALSE ("Visible")
            n191 = local read "DUD CAM"() -> (w299:T3)
            n192 = Index Array(array=w300) -> (element=w303:cluster{string[]})  [unwired: 1 in]
            n193 = Unbundle(w299) -> ("Frame Rate"=w298:i32, "Compression"=w297:i32, "Size"=w301:u16)
            n194 = Unbundle(w303) -> (w302:string[])
            n195 = Index Array(array=w302, index=w301) -> (element=w296:string)
            n196 = call-poly <vilib>:"Write Key.vi"("section"=w307, "value"=w296, "key"="Size", "refnum"=w292) -> ("refnum out"=w309:T19)  [unwired: 2 in, 5 out]
            n197 = call-poly <vilib>:"Write Key.vi"("section"=w307, "value"=w298, "key"="FrameRate", "refnum"=w309) -> ("refnum out"=w308:T19)  [unwired: 1 in, 6 out]
            n198 = property on="DUD CAM" class="Clust (strict)"("Visible"=w310) -> ()  [unwired: 2 in, 2 out]
            n199 = local write "DB Camera Config"(w310) -> ()
            n200 = call-poly <vilib>:"Write Key.vi"("section"=w307, "value"=w297, "key"="Compression", "refnum"=w308) -> ("refnum out"=w294:T19)  [unwired: 1 in, 6 out]
            n201 = call <vilib>:"Close Config Data.vi"("refnum"=w294) -> ("file path"=w295:path)  [unwired: 2 in, 8 out]
            n202 = call <vilib>:"Open Config Data.vi"("configuration file path"=w295) -> ("refnum"=w293:T19)  [unwired: 8 in, 2 out]
          }
          frame True {
            n203 = property on="DUD CAM" class="Clust (strict)"("Visible"=TRUE) -> ()  [unwired: 2 in, 2 out]
          }
        }
      }
      event "DUD CAM": Value Change {
        # "Update summary string when any elements of DB camera change"
        n204 = event-data() -> ("NewVal"=w324:T3)  [unwired: 1 in]
        n205 = Index Array(array=w320) -> (element=w319:cluster{string[]})  [unwired: 1 in]
        n206 = Unbundle(w324) -> ("Frame Rate"=w315:i32, "Compression"=w314:i32, "Size"=w317:u16)
        n207 = Unbundle(w319) -> (w318:string[])
        n208 = Index Array(array=w318, index=w317) -> (element=w316:string)
        n209 = Format Into String(format string="%s   %dfps   %d%%", w316, w315, w314) -> (resulting string=w321:string)  [unwired: 2 in, 1 out]
        n210 = Build Array(w321) -> (w322:string[])
        n211 = property on="DB Camera Config" class="Bool (strict)"("Strings [4]"=w322) -> ()  [unwired: 2 in, 2 out]
      }
      event "Motor.Enable": Value Change {
        # "When the test mode otor enable helper is set, update that\ntree row item's value"
        n212 = event-data() -> ("NewVal"=w330:bool)  [unwired: 1 in]
        n213 = Unbundle("Motor") -> ("Value"=w329:dbl)  [unwired: 1 out]
        n214 = Select(t=w329, s=w330, f=0.0) -> (s? t:f=w327:dbl)
        n215 = call <vilib>:"NT Write Number.vi"("Numeric"=w327, "Name"=w326) -> ()  [unwired: 9 in, 1 out]
      }
      event "Test Slider": Value Change {
        # "When the test mode slider helper is set, update that\ntree row item's value"
        n216 = event-data() -> ("NewVal"=w333:dbl)  [unwired: 1 in]
        n217 = call <vilib>:"NT Write Number.vi"("Numeric"=w333, "Name"=w334) -> ()  [unwired: 9 in, 1 out]
      }
      event "On/Off": Value Change {
        # "When the test mode on/off helper value is set, update that\ntree row item's value"
        n218 = event-data() -> ("NewVal"=w338:bool)  [unwired: 1 in]
        n219 = Boolean To (0,1)(Boolean=w338) -> (0, 1=w337:i16)
        n220 = call <vilib>:"NT Write Number.vi"("Numeric"=w337, "Name"=w336) -> ()  [unwired: 9 in, 1 out]
      }
      event "Rev/Fwd": Value Change {
        # "When the test mode helper value for relays is set, update that\ntree row item's value"
        n221 = event-data() -> ("NewVal.Forward"=w346:bool, "NewVal.Reverse"=w345:bool)  [unwired: 1 in]
        n222 = Boolean To (0,1)(Boolean=w346) -> (0, 1=w342:i16)
        n223 = Boolean To (0,1)(Boolean=w345) -> (0, 1=w344:i16)
        n224 = Negate(x=w344) -> (-x=w343:i16)
        n225 = Add(x=w342, y=w343) -> (x+y=w341:i16)
        n226 = call <vilib>:"NT Write Number.vi"("Numeric"=w341, "Name"=w340) -> ()  [unwired: 9 in, 1 out]
      }
      event "Test Ring": Value Change {
        # "When a test mode helper value is selected from the ring,\nset the tree item's variable to the string value"
        n227 = event-data() -> ("NewVal"=w350:u16)  [unwired: 1 in]
        n228 = property on="Test Ring" class="Ring (strict)"() -> ("Strings []"=w351:string[])  [unwired: 2 in, 2 out]
        n229 = Index Array(array=w351, index=w350) -> (element=w349:string)
        n230 = call <vilib>:"NT Write String.vi"("String"=w349, "Name"=w348) -> ()  [unwired: 9 in, 1 out]
      }
      event "Rec Mode": Value Change {
        # "Update globals for recording mode and path to read log from.\nClear when logging and let NetworkTables set path for vision to\nuse."
        n231 = event-data() -> ("NewVal"=w361:enum32{"Stop", "Record", "Playback"})  [unwired: 1 in]
        n232 = global write "WPI_DashboardLogging Global.vi" "Logging Filename"(path "") -> ()
        n233 = case shown="\"Playback\"" w361 {
          tunnel: w360 -> [_ w363 w371]
          tunnel: [_ _ w370] -> w357
          tunnel: [_ _ w369] -> _
          tunnel: w355 -> [_ _ w367]
          tunnel: cluster{i32, i32} {-250, 170} -> [_ _ w366]
          tunnel: [_ _ T22 {"Image Size"=TRUE, "Image Type"=TRUE, "Pixel Value"=TRUE, "ROI Information"=TRUE, "Zoom Factor"=FALSE} ("Image Information Shown:All Elements")] -> w353
          tunnel: [_ _ TRUE ("Zoom Factor")] -> w352
          frame Default {
          }
          frame "Stop", "Record" {
            # "Place Window too"
            n234 = invoke class="VI" method="FP.Close"(reference=w363) -> (reference out=w362:refnum<vi>)  [unwired: 2 in, 2 out]
            n235 = invoke class="VI" method="Abort VI"(reference=w362) -> ()  [unwired: 2 in, 3 out]
          }
          frame "Playback" {
            n236 = call "Open Playback Panel.vi"("Offset"=w366, "DB VI Ref"=w367, "Playback in"=w371) -> ("Playback out"=w368:refnum<vi>)  [unwired: 8 in]
            n237 = register-events(w368) -> (reference out=w370:refnum<event-registration>, error out=w369:errorcluster)  [unwired: 2 in]
          }
        }
        n238 = global write "WPI_DashboardLogging Global.vi" "Recording"(w361) -> ()
        n239 = property on="Camera Image" class="ImageControl"("Image Information Shown"=w353, "Image Information Visible"=w352) -> ()  [unwired: 2 in, 2 out]
        n240 = call <vilib>:"WPI_DashboardNT Log FieldName Cache.vi"("Operation"=enum16{"Lookup/Add", "Index", "Clear"}."Clear") -> ()  [unwired: 8 in, 3 out]
      }
      event Panel Close {
        w372 = enum32{"Stop", "Record", "Playback"}."Stop" ("Rec Mode")
        # "Playback window has been closed, abort"
        n241 = event-data() -> ()  [unwired: 1 in, 4 out]
        n242 = local write "Rec Mode"(w372) -> ()
        n243 = global write "WPI_DashboardLogging Global.vi" "Recording"(w372) -> ()
      }
      event Panel Close {
        # "Abort playback window and ourself"
        n244 = event-data() -> ()  [unwired: 1 in, 4 out]
        n245 = invoke class="VI" method="FP.Close"(reference=w377) -> (reference out=w376:refnum<vi>)  [unwired: 2 in, 2 out]
        n246 = invoke class="VI" method="Abort VI"(reference=w376) -> (error out=w375:errorcluster)  [unwired: 2 in, 2 out]
        n247 = invoke class="VI" method="Abort VI"(error in=w375) -> ()  [unwired: 2 in, 3 out]
      }
      event "Vision": Value Change {
        # "Enable/Disable Compression slider.\nHW USB is hard-coded into the camera"
        n248 = event-data() -> ("NewVal"=w383:u16)  [unwired: 1 in]
        n249 = Equal?(x=w383, y=u32 2 ("milliseconds to wait")) -> (x = y?=w381:bool)
        n250 = Select(t=T23."Disabled and Grayed Out" ("Disabled"), s=w381, f=T23."Enabled" ("Disabled")) -> (s? t:f=w378:T23)
        n251 = property on="Compression" class="Slide (strict)"("DisabledEnum"=w378) -> ()  [unwired: 2 in, 2 out]
      }
    }
  }
  n252 = while {
    tunnel: w45 -> [w386]
    i -> [w389]
    stop <- FALSE stop-if-true
    n253 = Wait (ms)(milliseconds to wait=u32 100) -> ()  [unwired: 1 out]
    n254 = case shown="\"Playback\"" "Rec Mode" {
      tunnel: w389 -> [_ _ w404]
      tunnel: [u32 2829099 ("Base Color") u32 11141120 ("Target Color") w393] -> w385
      frame "Stop", Default {
        # "Reset the color, extra updates don't cost much"
      }
      frame "Record" {
      }
      frame "Playback" {
        # "Playback"
        n255 = Quotient & Remainder(x=w404, y=u32 50 ("milliseconds to wait")) -> (x-y*floor(x/y)=w400:u32)  [unwired: 1 out]
        n256 = Divide(x=w400, y=u32 50 ("milliseconds to wait")) -> (x/y=w397:dbl)
        n257 = Multiply(x=6.283185307179586, y=w397) -> (x*y=w402:dbl)
        n258 = Sine(x=w402) -> (sin(x)=w401:dbl)
        n259 = Absolute Value(x=w401) -> (abs(x)=w394:dbl)
        n260 = call "Interpolate RGB Color.vi"("Proportion"=w394, "Target Color"=u32 30976, "Base Color"=u32 2829099) -> ("Result Color"=w393:u32)  [unwired: 8 in]
      }
    }
    n261 = property class="Pane"(reference=w386, "PaneColor"=w385) -> ()  [unwired: 1 in, 2 out]
  }
  n262 = TCP Create Listener(10:u16 1741 ("timeout ms (25000)")) -> (3:w9:refnum<k5>)  [unwired: 4 in, 2 out]
  n263 = while {
    tunnel: w9 -> [w406]
    stop <- FALSE stop-if-true
    n264 = TCP Wait On Listener(11:w406) -> (4:w405:refnum<k5>)  [unwired: 3 in, 4 out]
    n265 = local write "TCP"(w405) -> ()
  }
  n266 = property on="On/Off" class="Bool (strict)"("Visible"=w14) -> ()  [unwired: 2 in, 2 out]
  n267 = property on="Motor" class="Clust (strict)"("Visible"=w14) -> ()  [unwired: 2 in, 2 out]
  n268 = property on="Progress" class="Clust (strict)"("Visible"=w14) -> ()  [unwired: 2 in, 2 out]
  n269 = property on="Test Ring" class="Ring (strict)"("Visible"=w14) -> ()  [unwired: 2 in, 2 out]
  n270 = property on="Rev/Fwd" class="Clust (strict)"("Visible"=w14) -> ()  [unwired: 2 in, 2 out]
  n271 = property on="DUD CAM" class="Clust (strict)"("Visible"=w14) -> ()  [unwired: 2 in, 2 out]
  n272 = local write "DB Camera Config"(w14) -> ()
  n273 = global write "WPI_DashboardLogging Global.vi" "Recording"(w3) -> ()
  n274 = local write "Rec Mode"(w3) -> ()
  n275 = Tick Count (ms)() -> (millisecond timer value=w8:u32)
  n276 = while {
    tunnel: w8 -> [w410]
    stop <- FALSE stop-if-true
    n277 = Wait (ms)(milliseconds to wait=u32 1000) -> ()  [unwired: 1 out]
    n278 = call-poly <vilib>:"SD Read Value.vi"("Name"="Voltages" ("Table Prefix")) -> ("Numeric Array"=w428:dbl[])  [unwired: 8 in, 2 out]
    n279 = Tick Count (ms)() -> (millisecond timer value=w411:u32)
    n280 = Index Array(array=w428) -> (element #2=w427:dbl, element #3=w426:dbl, element #4=w425:dbl, element #5=w424:dbl, element #6=w423:dbl, element #7=w422:dbl, element #8=w421:dbl, element #9=w420:dbl, element #10=w419:dbl, element #11=w418:dbl, element #12=w417:dbl, element #13=w415:dbl, element #14=w416:dbl, element #15=w414:dbl, element #16=w413:dbl, element #17=w412:dbl)  [unwired: 17 in, 1 out]
    n281 = Subtract(x=w411, y=w410) -> (x-y=w409:u32)
    n282 = Build Array(w409, w427, w426, w425, w424, w423, w422, w421, w420, w419, w418, w417, w415, w416, w414, w413, w412) -> (w408:dbl[])
    n283 = case shown="True" "Export To File" {
      tunnel: "Save To" -> [_ w437]
      tunnel: w408 -> [_ w434]
      frame False {
      }
      frame True {
        n284 = call-poly <vilib>:"Write To Spreadsheet File.vi"("delimiter (\\t)"="," ("delimiter (\\t)"), "append to file? (new file:F)"=TRUE, "1D data"=w434, "file path (dialog if empty)"=w437) -> ()  [unwired: 4 in, 1 out]
      }
    }
  }
  n285 = call "IMAQ Create"("Image Name"="Dashboard Image", "Image Type"=w7) -> ("New Image"=w5:T1, "error out"=w4:errorcluster)  [unwired: 2 in, 1 out]
  n286 = call "IMAQ Create"("Image Name"="Dashboard Image 2", "Image Type"=w57) -> ("New Image"=w2:T1, "error out"=w1:errorcluster)  [unwired: 2 in, 1 out]
  n287 = while {
    tunnel: w5 -> [w459]
    tunnel: w4 -> [_]
    tunnel: [w460] -> _
    tunnel: w2 -> [w448]
    tunnel: w1 -> [_]
    i -> [w460]
    stop <- FALSE stop-if-true
    # "Optionally read the DB image,\nlog, or retrieve images from a\nlogged match"
    # "Optionally read the DB image,\nlog, or retrieve images from a\nlogged match"
    n288 = case shown="True" "CamPow" {
      tunnel: [w466 w468] -> w447
      tunnel: [w466 w467] -> w446
      frame False {
        w466 = u16 0 items=["Camera Off", "USB Camera SW", "USB Camera HW", "IP Camera"] ("Vision")
      }
      frame True {
        w467 = u16 1 items=["Camera Off", "USB Camera SW", "USB Camera HW", "IP Camera"] ("Vision")
        w468 = u16 3 items=["Camera Off", "USB Camera SW", "USB Camera HW", "IP Camera"] ("Vision")
      }
    }
    n289 = case shown="False" "Toggle View" {
      tunnel: [w462 w465] -> w441
      tunnel: "Big Cam" -> [w463 w465]
      tunnel: [w463 w464] -> w439
      tunnel: "Small Cam" -> [w462 w464]
      frame False {
      }
      frame True {
      }
    }
    n290 = local read "Camera Addr"() -> (w443:string)
    n291 = local read "Rec Mode"() -> (w454:enum32{"Stop", "Record", "Playback"})
    n292 = local read "Rec Mode"() -> (w453:enum32{"Stop", "Record", "Playback"})
    n293 = call <vilib>:"WPI_CameraRead MJPG for Dashboard.vi"("Camera Settings"=w441, "Rec Mode"=w454, "Camera IP"=w443, "Camera Mode"=w446, "Refnum in"=w459) -> ("Active"=w457:bool, "Refnum out"=w458:T1, "FPS"=w456:dbl, "Bandwidth (Mbps)"=w455:dbl)  [unwired: 3 in]
    n294 = call <vilib>:"WPI_CameraRead MJPG for Dashboard.vi"("Camera Settings"=w439, "Rec Mode"=w453, "Camera IP"="10.44.18.22", "Camera Mode"=w447, "Refnum in"=w448) -> ("Active"=w450:bool, "Refnum out"=w449:T1, "FPS"=w451:dbl, "Bandwidth (Mbps)"=w452:dbl)  [unwired: 3 in]
    n295 = case shown="True" w457 {
      tunnel: w458 -> [_ w491]
      tunnel: w455 -> [_ w490]
      tunnel: w456 -> [_ w489]
      tunnel: "Toggle View" -> [_ w486]
      frame False {
        # "Sleep for 500ms"
        n296 = Wait Until Next ms Multiple(millisecond multiple=u32 500) -> ()  [unwired: 1 out]
      }
      frame True {
        # "Here is where you would annotate,\npossibly process, and display the image"
        # "Update Mbps LED"
        n297 = call "IMAQ Clear Overlay"("Image"=w491) -> ("error out"=w494:errorcluster, "Image Out"=w487:T1)  [unwired: 2 in, 7 out]
        n298 = case shown="4, 5" w490 {
          tunnel: [u32 6618880 ("Color Box") u32 16776722 ("Color Box") u32 16716800 ("Color Box")] -> w492
          frame Default {
          }
          frame 4, 5 {
          }
          frame 6.. {
          }
        }
        n299 = Unbundle By Name(w494) -> ("status"=w495:bool)
        n300 = Bundle("Color Box"=w492, "Color Box"=w492) -> (w493:cluster{"Color Box":u32, "Color Box":u32})  [unwired: 1 out]
        n301 = property on="Image Message" class="Str"("Visible"=w495) -> ()  [unwired: 2 in, 2 out]
        n302 = Build Array(w493) -> (w488:cluster{"Color Box":u32, "Color Box":u32}[])
        n303 = property on="Mbps 4" class="Bool (strict)"("Colors [4]"=w488) -> ()  [unwired: 2 in, 2 out]
        n304 = case shown="False" w486 {
          tunnel: w487 -> [w496 w497]
          frame False {
            n305 = local write "Camera Image 2"(w496) -> ()
          }
          frame True {
            n306 = local write "Camera Image"(w497) -> ()
          }
        }
        "Mbps 3" <- w490
        "fps 2" <- w489
      }
    }
    n307 = case shown="True" w450 {
      tunnel: w449 -> [_ w474]
      tunnel: w452 -> [_ w473]
      tunnel: w451 -> [_ w472]
      tunnel: "Toggle View" -> [_ w470]
      frame False {
        # "Sleep for 500ms"
        n308 = Wait Until Next ms Multiple(millisecond multiple=u32 500) -> ()  [unwired: 1 out]
      }
      frame True {
        # "Here is where you would annotate,\npossibly process, and display the image"
        # "Update Mbps LED"
        n309 = call "IMAQ Clear Overlay"("Image"=w474) -> ("error out"=w478:errorcluster, "Image Out"=w471:T1)  [unwired: 2 in, 7 out]
        n310 = case shown="4, 5" w473 {
          tunnel: [u32 6618880 ("Color Box") u32 16776722 ("Color Box") u32 16716800 ("Color Box")] -> w475
          frame Default {
          }
          frame 4, 5 {
          }
          frame 6.. {
          }
        }
        n311 = Unbundle By Name(w478) -> ("status"=w479:bool)
        n312 = Bundle("Color Box"=w475, "Color Box"=w475) -> (w477:cluster{"Color Box":u32, "Color Box":u32})  [unwired: 1 out]
        n313 = property on="Image Message" class="Str"("Visible"=w479) -> ()  [unwired: 2 in, 2 out]
        n314 = Build Array(w477) -> (w476:cluster{"Color Box":u32, "Color Box":u32}[])
        n315 = property on="Mbps 2" class="Bool (strict)"("Colors [4]"=w476) -> ()  [unwired: 2 in, 2 out]
        n316 = case shown="False" w470 {
          tunnel: w471 -> [w480 w481]
          frame False {
            n317 = local write "Camera Image"(w480) -> ()
          }
          frame True {
            n318 = local write "Camera Image 2"(w481) -> ()
          }
        }
        "Mbps" <- w473
        "fps" <- w472
      }
    }
  }
